vi "gotoTopBotExp2.vi"(8 "error in (no error)":errorcluster, 9 "position":refnum<vi>, 10 "motor setting":refnum<vi>, 11 "appended array":refnum<k7>[](array[refnum])) -> (0 "error out":errorcluster)   [LabVIEW 2014]
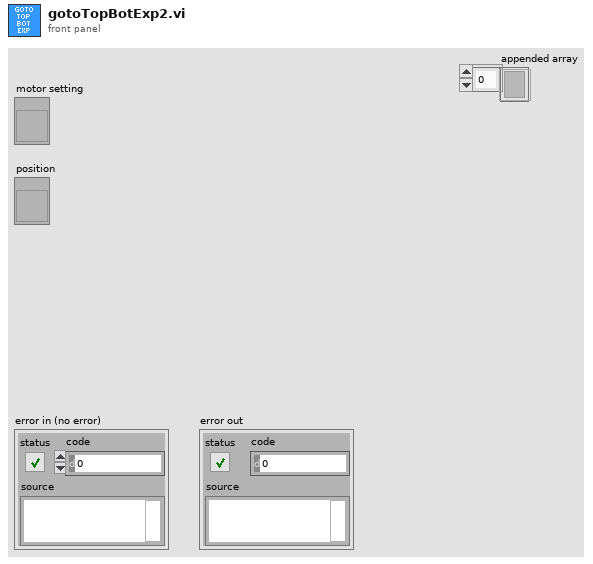
[diagram p1: front panel]
types:
  T1 = cluster{"X Acc (mm/s^2)":sgl, "X Vmax (mm/s)":sgl, "Y Acc (mm/s^2)":sgl, "Y Vmax (mm/s)":sgl, "Z Acc (mm/s^2)":sgl, "Z Vmax (mm/s)":sgl}
  T2 = cluster{"X Pos (mm)":sgl, "Y Pos (mm)":sgl, "Z Pos (mm)":sgl}
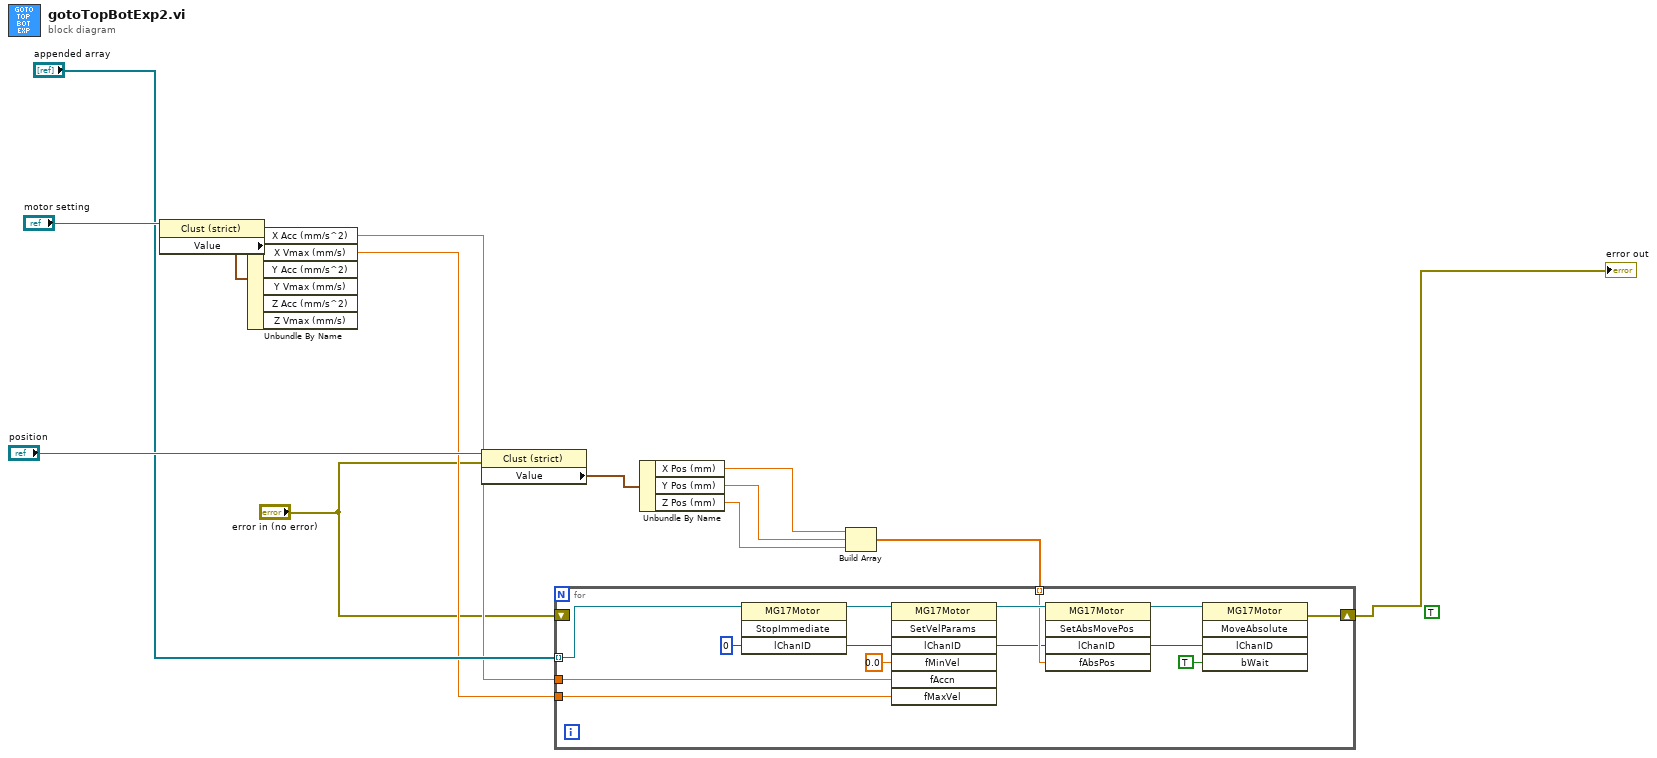
[diagram p0: block diagram]
diagram:
  (unwired) TRUE
  n1 = property on="Property Node" class="Clust (strict)"(reference="motor setting") -> ("Value"=w8:T1)  [unwired: 1 in, 2 out]
  n2 = Unbundle By Name(w8) -> ("X Acc (mm/s^2)"=w6:sgl, "X Vmax (mm/s)"=w7:sgl)  [unwired: 4 out]
  n3 = property on="Property Node" class="Clust (strict)"(reference="position", error in="error in (no error)") -> ("Value"=w9:T2)  [unwired: 2 out]
  n4 = Unbundle By Name(w9) -> ("X Pos (mm)"=w5:sgl, "Y Pos (mm)"=w4:sgl, "Z Pos (mm)"=w3:sgl)
  n5 = Build Array(w5, w4, w3) -> (w2:sgl[])
  n6 = for {
    tunnel: "appended array" -> [w27] mode=indexing
    tunnel: w7 -> [w21]
    tunnel: w6 -> [w20]
    tunnel: w2 -> [w17] mode=indexing
    shift-right: [w16] -> w13
    shift-left: "error in (no error)" -> [_]
    n7 = invoke class="MG17Motor" method="StopImmediate"(reference=w27, "lChanID"=0) -> (reference out=w26:refnum<k7>, "lChanID"=w15:i32)  [unwired: 2 in, 2 out]
    n8 = invoke class="MG17Motor" method="SetVelParams"(reference=w26, "lChanID"=w15, "fMinVel"=sgl 0.0, "fAccn"=w20, "fMaxVel"=w21) -> (reference out=w25:refnum<k7>, "lChanID"=w14:i32)  [unwired: 2 in, 5 out]
    n9 = invoke class="MG17Motor" method="SetAbsMovePos"(reference=w25, "lChanID"=w14, "fAbsPos"=w17) -> (reference out=w24:refnum<k7>, "lChanID"=w19:i32)  [unwired: 2 in, 3 out]
    n10 = invoke class="MG17Motor" method="MoveAbsolute"(reference=w24, "lChanID"=w19, "bWait"=TRUE) -> (error out=w16:errorcluster)  [unwired: 2 in, 4 out]
  }
  "error out" <- w13
